vi "Hatch Call.vi"(9 "Call Context":T1, 10 "Left Button Values":bool[](array[boolean])) -> ()   [LabVIEW 2018]
uses:
  <vilib>/Rock Robotics/WPI/DriverStation/WPI_DriverStationDerivedRobotMode.ctl
  Implementation/Hatch Setpoints.ctl
  Implementation/Hatch Operations.ctl
  <vilib>/Rock Robotics/Network Tables/NT Write Boolean.vi
  <vilib>/functionblocks/Edge Detection/One Shot Falling With Input/One Shot Falling With Input.vi
  <vilib>/functionblocks/Edge Detection/One Shot Rising with Input/One Shot Rising with Input.vi
  <vilib>/functionblocks/FB Core/FB Core.xnode
  <vilib>/functionblocks/NI_FunctionBlock Libraries.lvlib
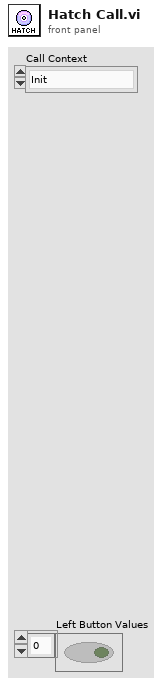
[diagram p1: front panel]
types:
  T1 = typedef "WPI_DriverStationDerivedRobotMode.ctl" = enum16{"Init", "Execute", "Stop"}
  T2 = typedef "Hatch Setpoints.ctl" = cluster{"Operation":T3}
  T3 = typedef "Hatch Operations.ctl" = enum16{"Reserve", "Read Current", "Hatch Gripper In", "Hatch Gripper Out", "Extend Gripper Plate", "Retract Gripper Plate", "Retract HAB Piston", "Extend HAB Piston"}
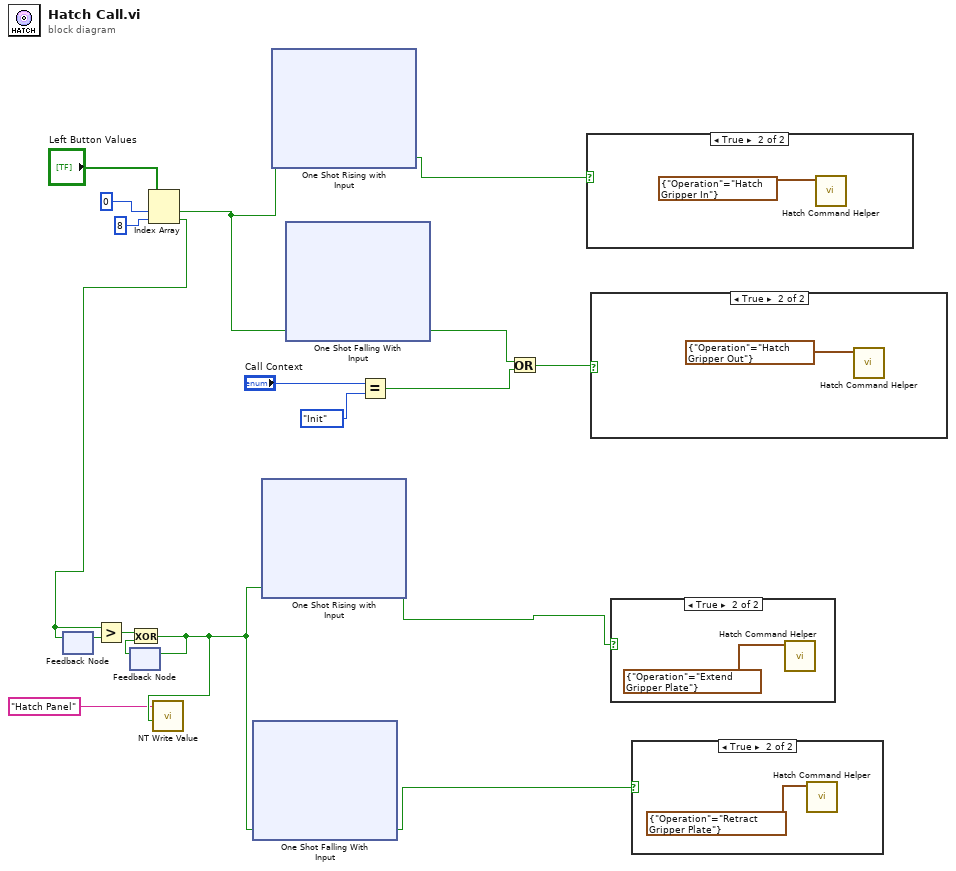
[diagram p0: block diagram]
diagram:
  n1 = feedback #1() -> (w9:bool)  [unwired: 1 in]
  n2 = feedback #2() -> (w7:bool)  [unwired: 1 in]
  n3 = Index Array(array="Left Button Values", index #1=0 ("index"), index #2=8 ("index")) -> (element #1=w17:bool, element #2=w6:bool)
  n4 = feedback-in #1(w6) -> ()
  n5 = Greater?(x=w6, y=w9) -> (0:w8:bool)
  n6 = Exclusive Or(1:w7, 2:w8) -> (0:w5:bool)
  n7 = feedback-in #2(w5) -> ()
  n8 = call-poly <vilib>:"NT Write Value.vi"("Boolean"=w5, "Name"="Hatch Panel") -> ()  [unwired: 9 in, 1 out]
  n9 = xnode "One Shot Falling With Input"("input"=w5) -> ("output"=w3:bool)  [unwired: 1 in, 1 out]
  n10 = xnode "One Shot Rising with Input"("input"=w5) -> ("output"=w2:bool)  [unwired: 1 in, 1 out]
  n11 = xnode "One Shot Rising with Input"("input"=w17) -> ("output"=w16:bool)  [unwired: 1 in, 1 out]
  n12 = xnode "One Shot Falling With Input"("input"=w17) -> ("output"=w14:bool)  [unwired: 1 in, 1 out]
  n13 = Equal?(x="Call Context", y=WPI_DriverStationDerivedRobotMode."Init") -> (x = y?=w1:bool)
  n14 = Or(x=w14, y=w1) -> (x .or. y?=w15:bool)
  n15 = case shown="True" w16 {
    frame False {
    }
    frame True {
      n16 = call "Hatch Command Helper.vi"("SubSystem Data"=T2 {"Operation"=enum."Hatch Gripper In"}) -> ()  [unwired: 8 in, 3 out]
    }
  }
  n17 = case shown="True" w15 {
    frame False {
    }
    frame True {
      n18 = call "Hatch Command Helper.vi"("SubSystem Data"=T2 {"Operation"=enum."Hatch Gripper Out"}) -> ()  [unwired: 8 in, 3 out]
    }
  }
  n19 = case shown="True" w2 {
    frame False {
    }
    frame True {
      n20 = call "Hatch Command Helper.vi"("SubSystem Data"=T2 {"Operation"=enum."Extend Gripper Plate"}) -> ()  [unwired: 8 in, 3 out]
    }
  }
  n21 = case shown="True" w3 {
    frame False {
    }
    frame True {
      n22 = call "Hatch Command Helper.vi"("SubSystem Data"=T2 {"Operation"=enum."Retract Gripper Plate"}) -> ()  [unwired: 8 in, 3 out]
    }
  }
